vi "finishKickoffAllyPlayVSS.vi"(8 "error in (no error)":errorcluster, 10 "Game in":refnum<class "Game.lvclass">, 11 "KickoffAllyPlayVSS in":refnum<class "KickoffAllyPlayVSS.lvclass">) -> (0 "error out":errorcluster, 2 "result":bool, 3 "KickoffAllyPlayVSS out":refnum<class "KickoffAllyPlayVSS.lvclass">)   [LabVIEW 2020, in "KickoffAllyPlayVSS.lvclass"]
uses:
  KickoffAllyPlayVSS.lvclass
  Game_class/Game.lvclass
  Game_class/Game.lvclass/Game.ctl
  Events_class/Events.lvclass/Events.ctl
  Game_class/Read Referee.vi
  Game_class/Read EventsRef.vi
  Events_class/Read ball_out.vi
  Events_class/Read touch.vi
  Events_class/Read id_touch.vi
  Referee_class/Referee.lvclass
  Events_class/Events.lvclass
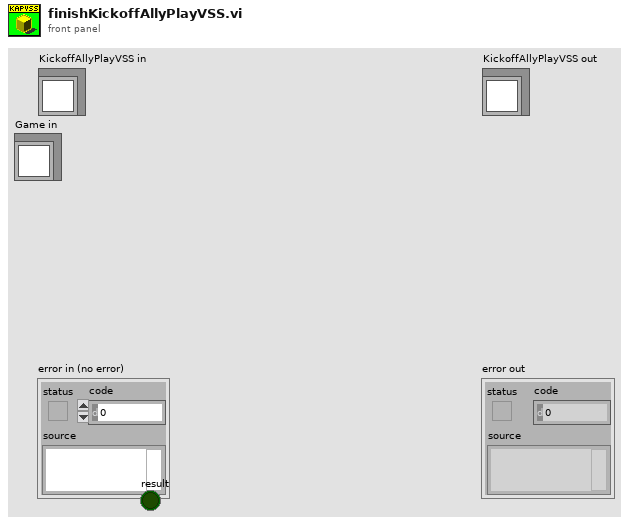
[diagram p1: front panel]
types:
  T1 = enum16{"AUTO", "GAME_ON", "STOP", "KICKOFF", "FREE_BALL", "GOAL_KICK", "PENALTY_KICK", "FREE_KICK"}
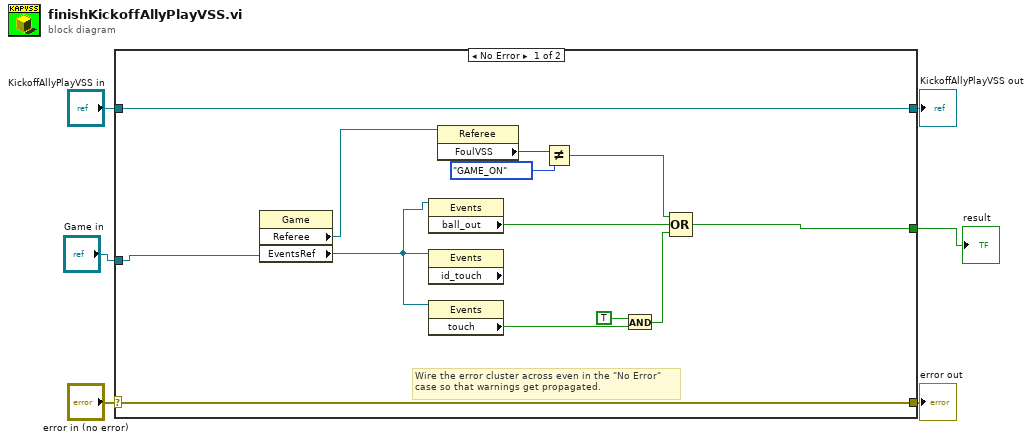
[diagram p0: block diagram]
diagram:
  n1 = case shown="No Error" "error in (no error)" {
    selector: "error in (no error)" -> [w18 w21]
    tunnel: [w18 w21] -> w5
    tunnel: [w19 w20] -> w3
    tunnel: "KickoffAllyPlayVSS in" -> [w19 w20]
    tunnel: "Game in" -> [w12 _]
    tunnel: [w11 _] -> w1
    frame No Error {
      # "Wire the error cluster across even in the \"No Error\"\ncase so that warnings get propagated."
      n2 = property class="Game"(reference=w12) -> ("Referee"=w8:refnum<class "Referee.lvclass">, "EventsRef"=w14:refnum<class "Events.lvclass">)  [unwired: 1 in, 2 out]
      n3 = property class="Events"(reference=w14) -> ("ball_out"=w17:bool)  [unwired: 1 in, 2 out]
      n4 = property class="Events" props=["id_touch"](reference=w14) -> ()  [unwired: 1 in, 3 out]
      n5 = property class="Events"(reference=w14) -> ("touch"=w15:bool)  [unwired: 1 in, 2 out]
      n6 = property class="Referee"(reference=w8) -> ("FoulVSS"=w10:T1)  [unwired: 1 in, 2 out]
      n7 = Not Equal?(x=w10, y=T1."GAME_ON") -> (x != y?=w7:bool)
      n8 = And(x=TRUE, y=w15) -> (x .and. y?=w16:bool)
      n9 = Compound Arithmetic op=OR(w7, w17, w16) -> (w11:bool)
    }
    frame Error {
    }
  }
  "error out" <- w5
  "KickoffAllyPlayVSS out" <- w3
  "result" <- w1
